vi "Simulated Speaker.vi"() -> ()   [LabVIEW 2010]
uses:
  <vilib>/DAQmx/read.llb/DAQmx Read (Analog Wfm 1Chan NSamp).vi
  <vilib>/DAQmx/create/channels.llb/DAQmx Create Channel (AI-Voltage-Basic).vi
  <vilib>/DAQmx/configure/timing.llb/DAQmx Timing (Sample Clock).vi
  <vilib>/DAQmx/configure/trigger.llb/DAQmx Start Trigger (Digital Edge).vi
  Instance          10 25Saved   Simulated Speaker .vi
  <vilib>/daqmx/miscellaneous.llb/DAQmx Fill In Error Info.vi
panel:
  out "Mono-Channel Sound Signal":waveform(dbl)(graph)={"t0"=timestamp(6.792281999999995 s since 1904-01-01), "dt"=2.264999999999998e-05, "Y"=array[8820 elements], "attributes"=variant("NI_ChannelName"=variant(string "cDAQ1Mod2/ai3"), "NI_UnitDescription"=variant(string "Volts"))}
  in  "physical channels":tag="cDAQ1Mod2/ai3"
  in  "Sample Rate":dbl=44100.0 format="%0.2f"
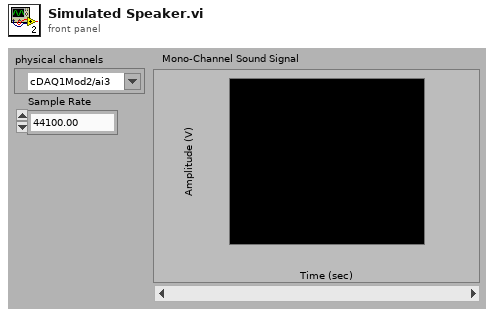
[diagram p1: front panel]
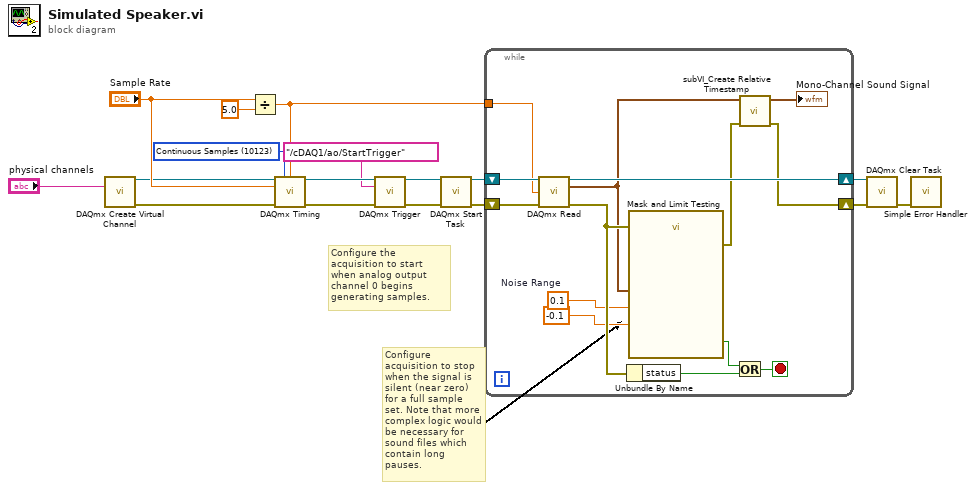
[diagram p0: block diagram]
diagram:
  w15 = 10123 items=["Finite Samples"=10178, "Continuous Samples"=10123, "Hardware Timed Single Point"=12522] ("sample mode")
  # "Configure the acquisition to start when analog output channel 0 begins generating samples."
  # "Configure acquisition to stop when the signal is silent (near zero) for a full sample set. Note that more complex logic would be necessary for sound files which contain long pauses."
  n1 = call-poly <vilib>:"DAQmx Create Virtual Channel.vi"("physical channels"="physical channels") -> ("task out"=w5:refnum<k21>, "error out"=w4:errorcluster)  [unwired: 13 in]
  n2 = Divide(x="Sample Rate", y=5.0) -> (x/y=w13:dbl)
  n3 = call-poly <vilib>:"DAQmx Timing.vi"("task/channels in"=w5, "sample mode"=w15, "samples per channel"=w13, "rate"="Sample Rate", "error in"=w4) -> ("task out"=w16:refnum<k21>, "error out"=w17:errorcluster)  [unwired: 9 in]
  n4 = call-poly <vilib>:"DAQmx Trigger.vi"("task/channels in"=w16, "source"=tag "/cDAQ1/ao/StartTrigger", "error in"=w17) -> ("task out"=w10:refnum<k21>, "error out"=w8:errorcluster)  [unwired: 11 in]
  n5 = call <vilib>:"DAQmx Start Task.vi"("task/channels in"=w10, "error in"=w8) -> ("task out"=w9:refnum<k21>, "error out"=w7:errorcluster)  [unwired: 12 in]
  n6 = while {
    tunnel: w13 -> [w25]
    shift-right: [w20] -> w11
    shift-left: w7 -> [w30]
    shift-right: [w24] -> w12
    shift-left: w9 -> [w31]
    stop <- w26 stop-if-true
    w19 = 0.1  # Noise Range
    n7 = call-poly <vilib>:"DAQmx Read.vi"("task/channels in"=w31, "number of samples per channel"=w25, "error in"=w30) -> ("task out"=w24:refnum<k21>, "data"=w22:waveform(dbl), "error out"=w29:errorcluster)  [unwired: 10 in]
    n8 = Unbundle By Name(w29) -> ("status"=w27:bool)
    n9 = call "Mask and Limit Testing"("Lower Constant"=-0.1 ("window bottom"), "Upper Constant"=w19, "error in"=w29, "Signals"=w22) -> ("error out"=w21:errorcluster, "Passed"=w28:bool)  [unwired: 4 in, 2 out]
    n10 = Or(x=w28, y=w27) -> (x .or. y?=w26:bool)
    n11 = call "subVI_Create Relative Timestamp.vi"("error in (no error)"=w21, "waveform in"=w22) -> ("error out"=w20:errorcluster, "waveform out"=→"Mono-Channel Sound Signal":waveform(dbl))  [unwired: 8 in]
  }
  n12 = call <vilib>:"DAQmx Clear Task.vi"("task in"=w12, "error in"=w11) -> ("error out"=w1:errorcluster)  [unwired: 13 in]
  n13 = call <vilib>:"Simple Error Handler.vi"("error in (no error)"=w1) -> ()  [unwired: 4 in, 5 out]
